vi "test_dragon_file--read_project_settings.vi"(8 "error in (no error)":errorcluster) -> (0 "error out":errorcluster)   [LabVIEW 2020]
uses:
  906ee365-77ae-4f67-adba-29ffbc9f450d.vi
  906ee365-77ae-4f67-adba-29ffbc9f450d.vi/05157253-4ade-4b75-9902-c642c5dd4762.vi
  906ee365-77ae-4f67-adba-29ffbc9f450d.vi/543db544-a529-4041-9332-0fe0cbee0c9f.vi
  toml/read_subtable_key_string.vi
  toml/toml.lvclass
  <vilib>/addons/_JKI Toolkits/Caraya/classes/Assert/Assert.lvclass
  <vilib>/addons/_JKI Toolkits/Caraya/classes/Test/Test.lvclass
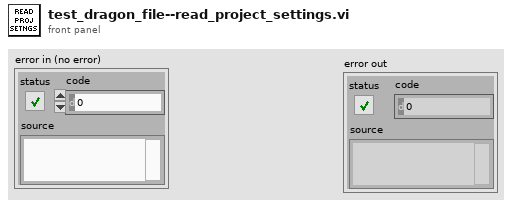
[diagram p1: front panel]
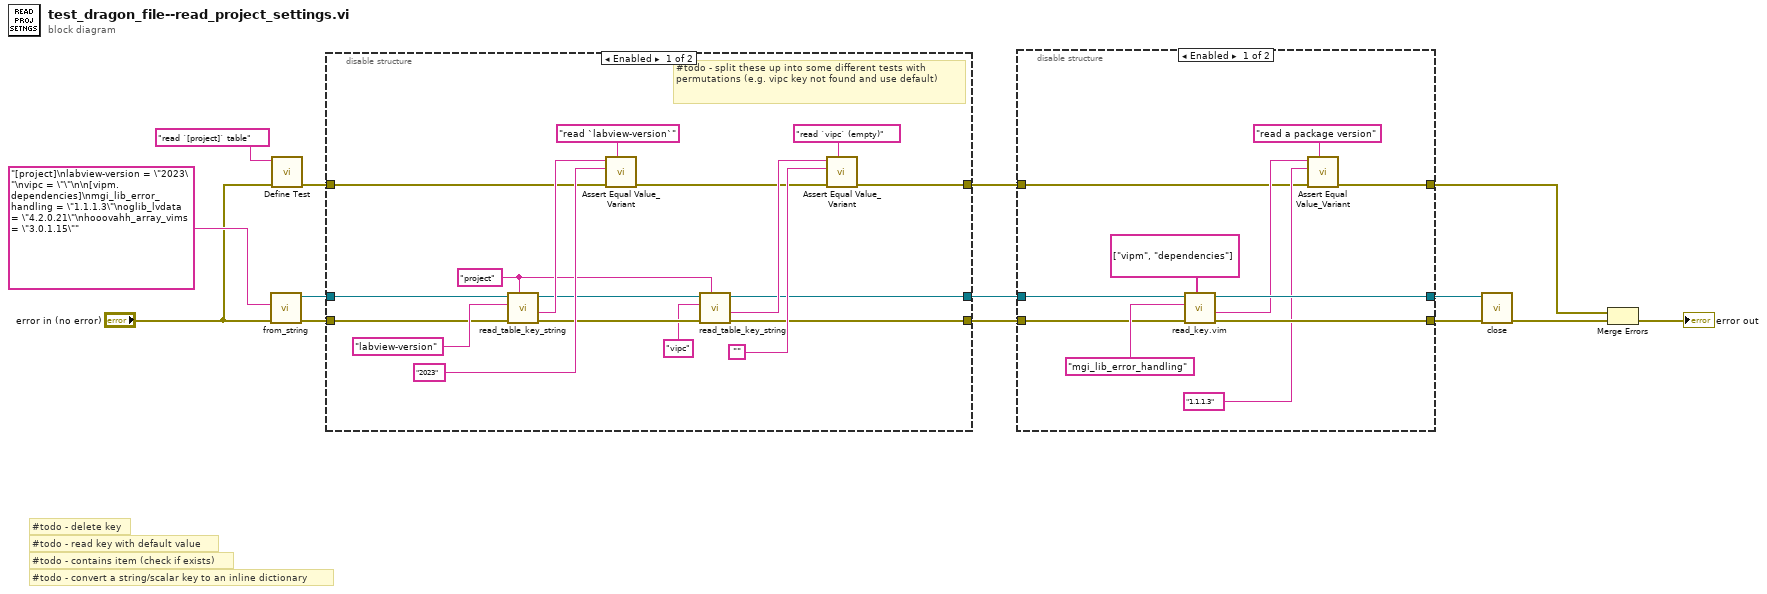
[diagram p0: block diagram]
diagram:
  # "#todo - contains item (check if exists)"
  # "#todo - convert a string/scalar key to an inline dictionary"
  # "#todo - read key with default value"
  # "#todo - delete key"
  n1 = call "from_string.vi"("error in (no error)"="error in (no error)", "toml"="[project]\nlabview-version = \"2023\"\nvipc = \"\"\n\n[vipm.dependencies]\nmgi_lib_error_handling = \"1.1.1.3\"\noglib_lvdata = \"4.2.0.21\"\nhooovahh_array_vims = \"3.0.1.15\"" ("toml_string in")) -> ("error out"=w8:errorcluster, "toml out"=w9:refnum<class "toml.lvclass">)  [unwired: 8 in]
  n2 = call <vilib>:"Define Test.vi"("error in (no error)"="error in (no error)", "Label (VI Title)"="read `[project]` table") -> ("error out"=w11:errorcluster)  [unwired: 9 in]
  n3 = disable-structure "Diagram Disable Structure" shown="Enabled" {
    disable-tunnel: w11 -> [w28 w33]
    disable-tunnel: w9 -> [w27 w35]
    disable-tunnel: w8 -> [w26 w34]
    disable-tunnel: [w18 w33] -> w3
    disable-tunnel: [w17 w34] -> w2
    disable-tunnel: [w16 w35] -> w1
    frame Enabled {
      w15 = "project" ("table_name")
      # "#todo - split these up into some different tests with permutations (e.g. vipc key not found and use default)"
      n4 = call "read_table_key_string.vi"("table"=w15, "error in (no error)"=w26, "key"="labview-version" ("table_name"), "toml in"=w27) -> ("error out"=w24:errorcluster, "value"=w31:string, "toml out"=w25:refnum<class "toml.lvclass">)  [unwired: 4 in, 1 out]
      n5 = call <vilib>:"Assert Equal Value_Variant.vi"("Label"="read `labview-version`", "error in (no error)"=w28, "Y"="2023" ("string"), "X"=w31) -> ("error out"=w19:errorcluster)  [unwired: 7 in]
      n6 = call "read_table_key_string.vi"("table"=w15, "error in (no error)"=w24, "key"="vipc" ("table_name"), "toml in"=w25) -> ("error out"=w17:errorcluster, "value"=w21:string, "toml out"=w16:refnum<class "toml.lvclass">)  [unwired: 4 in, 1 out]
      n7 = call <vilib>:"Assert Equal Value_Variant.vi"("Label"="read `vipc` (empty)", "error in (no error)"=w19, "Y"="" ("table_name"), "X"=w21) -> ("error out"=w18:errorcluster)  [unwired: 7 in]
    }
    frame Disabled {
    }
  }
  n8 = disable-structure "Diagram Disable Structure" shown="Enabled" {
    disable-tunnel: [w45 w49] -> w6
    disable-tunnel: [w44 w48] -> w5
    disable-tunnel: [w39 w47] -> w4
    disable-tunnel: w3 -> [w38 w47]
    disable-tunnel: w2 -> [w37 w48]
    disable-tunnel: w1 -> [w36 w49]
    frame Enabled {
      n9 = call "read_key.vim"("table"=string[] ["vipm", "dependencies"], "error in (no error)"=w37, "key"="mgi_lib_error_handling" ("table_name"), "toml in"=w36) -> ("error out"=w44:errorcluster, "value"=w41:string, "toml out"=w45:refnum<class "toml.lvclass">)  [unwired: 4 in, 1 out]
      n10 = call <vilib>:"Assert Equal Value_Variant.vi"("Label"="read a package version", "error in (no error)"=w38, "Y"="1.1.1.3" ("table_name"), "X"=w41) -> ("error out"=w39:errorcluster)  [unwired: 7 in]
    }
    frame Disabled {
    }
  }
  n11 = call "close.vi"("error in (no error)"=w5, "toml in"=w6) -> ("error out"=w7:errorcluster)  [unwired: 9 in]
  n12 = Merge Errors(w4, w7) -> (→"error out":errorcluster)
